vi "Find Tests - When Project Contains Theory - Returns Test Cases With Qualified Name.vi"() -> ()   [LabVIEW 2017, in "LVUnit Test Discoverer.Tests.lvlib"]
uses:
  LVUnit Test Discoverer.Tests.lvlib
  LVUnit Test Discoverer/LVUnit Test Discoverer.lvclass
  Test Case/Test Case.lvclass/Test Case.ctl
  Test Case/Get Qualified Name.vi
  03f621dc-86fc-49f7-a752-36e5275b9752.vi
  <vilib>/PNR/Transparent Assertions/Transparent Assertions/Constraints/IsEqual/Create.vi
  <vilib>/PNR/Transparent Assertions/Transparent Assertions/Constraints/IsEqual/IsEqual.lvclass
  Test Case/Test Case.lvclass
panel:
  out "error out":errorcluster
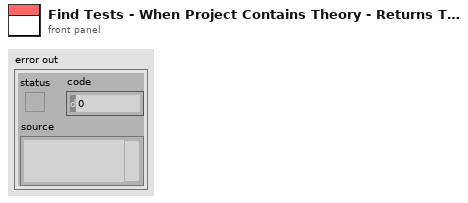
[diagram p1: front panel]
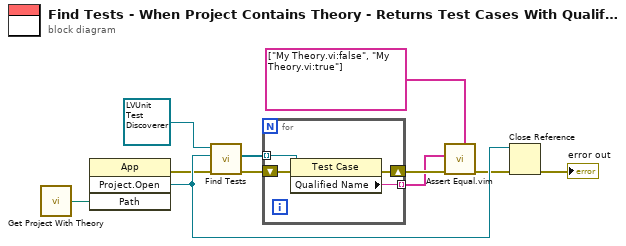
[diagram p0: block diagram]
diagram:
  n1 = call "Get Project With Theory.vi"() -> ("Project File"=w6:path)  [unwired: 2 in]
  n2 = invoke class="App" method="Project.Open"("Path"=w6) -> (error out=w7:errorcluster, "Project:Open"=w8:refnum<vi>)  [unwired: 3 in, 2 out]
  n3 = call-dynamic "Find Tests.vi"("error in (no error)"=w7, "Project Refnum"=w8, "LVUnit Test Discoverer in"=refnum<class "LVUnit Test Discoverer.lvclass"> refnum ("LVUnit Test Discoverer")) -> ("error out"=w10:errorcluster, "Test Cases"=w2:refnum<class "Test Case.lvclass">[])  [unwired: 6 in, 1 out]
  n4 = for {
    tunnel: [w13] -> w3 mode=indexing
    shift-right: [w14] -> w5
    shift-left: w10 -> [w15]
    tunnel: w2 -> [w12] mode=indexing
    n5 = property class="Test Case"(reference=w12, error in=w15) -> (error out=w14:errorcluster, "Qualified Name"=w13:string)  [unwired: 1 out]
  }
  n6 = call "Assert Equal.vim"("Expected"=string[] ["My Theory.vi:false", "My Theory.vi:true"], "error in (no error)"=w5, "Actual"=w3) -> ("error out"=w4:errorcluster)  [unwired: 8 in]
  n7 = Close Reference(reference=w8, error in (no error)=w4) -> (error out=→"error out":errorcluster)
